vi "MailDemo(冲突时的文件备份2013-03-27 14-08-18).vi"() -> ()   [LabVIEW 2012, in "Email.lvclass"]
uses:
  Email.lvclass
  MailInfo.ctl
  CredencialInfo.ctl
panel:
  out "error out":errorcluster caption="错误输出"
  in  "验证邮箱":T1={"邮件服务器（Host）"="smtp.126.com", "用户名"="csxcs_366", "密码"="******************************************"}
  in  "邮件信息":T2={"发送者地址"="csxcs_366@126.com", "发送者姓名"="陈树学", "接收者地址"=["276509891@qq.com"], "邮件主题"="测试邮件", "邮件内容"="该邮件仅用于发送邮件测试，接收后请删除。", "添加附件"=[path "E:/符号/状态图/接线端.png"]}
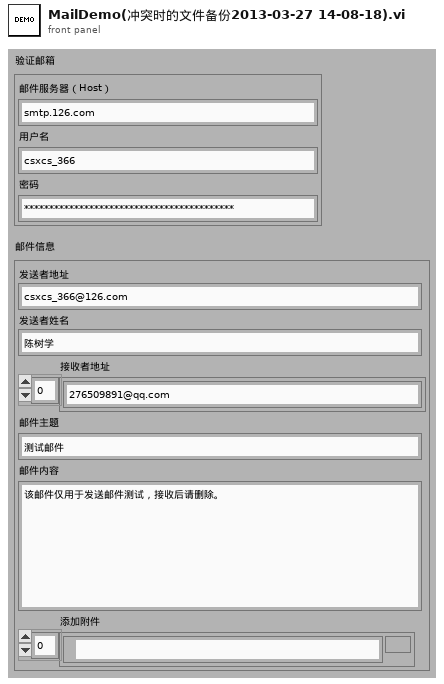
[diagram p1: front panel]
types:
  T1 = typedef "Email.lvclass/CredencialInfo.ctl" = cluster{"邮件服务器（Host）":string, "用户名":string, "密码":string}
  T2 = typedef "Email.lvclass/MailInfo.ctl" = cluster{"发送者地址":string, "发送者姓名":string, "接收者地址":string[], "邮件主题":string, "邮件内容":string, "添加附件":path[]}
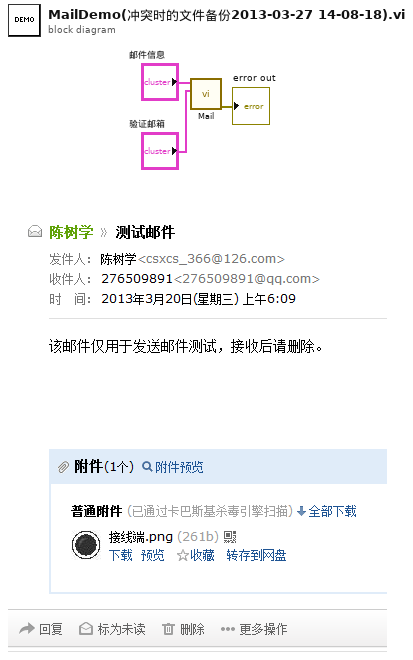
[diagram p0: block diagram]
diagram:
  n1 = call "Mail.vi"("验证邮箱"="验证邮箱", "邮件信息"="邮件信息") -> ("error out"=→"error out":errorcluster)  [unwired: 8 in, 1 out]
